vi "Auto Choose Resource.vi"(8 "error in (no error)":errorcluster, 11 "RP2040Target in":refnum<class "RP2040Target.lvclass">) -> (0 "error out":errorcluster, 1 "Cancelled":bool, 2 "Resource":refnum<class "DeployResource.lvclass">, 3 "RP2040Target out":refnum<class "RP2040Target.lvclass">)   [LabVIEW 2020, in "RP2040.lvlib" / "RP2040Target.lvclass"]
uses:
  RP2040Target.lvclass
  Builds/picoG/ppl/PicoG-Core.lvlibp/DeployResource/DeployResource.lvclass
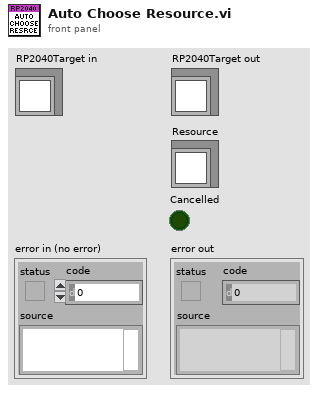
[diagram p1: front panel]
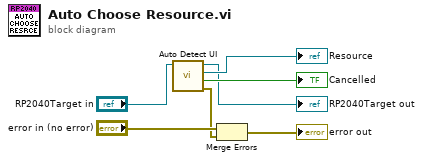
[diagram p0: block diagram]
diagram:
  n1 = call "Auto Detect UI.vi"("RP2040Target in"="RP2040Target in") -> ("error out"=w1:errorcluster, "Cancelled"=→"Cancelled":bool, "Resource"=→"Resource":refnum<class "DeployResource.lvclass">, "RP2040Target out"=→"RP2040Target out":refnum<class "RP2040Target.lvclass">)  [unwired: 7 in]
  n2 = Merge Errors("error in (no error)", w1) -> (→"error out":errorcluster)
